vi "Send.vi"(8 "error in":errorcluster, 11 "Block Upload Initiate in":refnum<class "Block Upload Initiate Transfer.lvclass">) -> (0 "error out":errorcluster, 3 "Block Upload Initiate out":refnum<class "Block Upload Initiate Transfer.lvclass">)   [LabVIEW 2020, in "CANopen.lvlib" / "SDO Manager.lvlib" / "Block Upload Initiate Transfer.lvclass"]
doc: "SDO block upload initiate (phase I)"
uses:
  Block Upload Initiate Transfer.lvclass
  D:/git/CANopen-LabVIEW/source/SDO/SDO Manager/SDO Transfer/SDO Transfer.lvclass
  Typedefs/Function Code.ctl
  SDO Transfer/SDO Transfer.lvclass/SDO Transfer.ctl
  Block Upload Initiate Transfer.lvclass/Block Upload Initiate Transfer.ctl
  CANopen Message/CANopen Message.lvclass/CANopen Message.ctl
  SDO Transfer/Get ICommunicate.vi
  SDO Transfer/Get Node-ID.vi
  SDO Transfer/Get Multiplexer.vi
  Get Block Size.vi
  Get Protocol Switch Threshold.vi
  CANopen Message/Encode COB-ID.vi
  HAL/Source/Interfaces/ICommunicate/ICommunicate.lvclass
  CANopen Message/CANopen Message.lvclass
  CANopen.lvlib
  SDO Transfer/SDO Transfer.lvclass
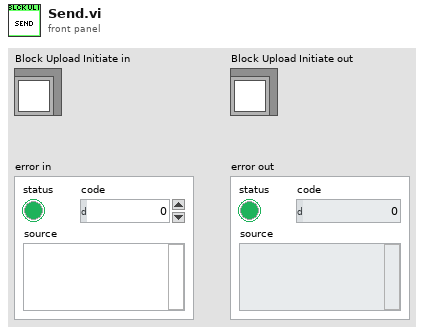
[diagram p1: front panel]
types:
  T1 = typedef "CANopen.lvlib/Function Code.ctl" = u8
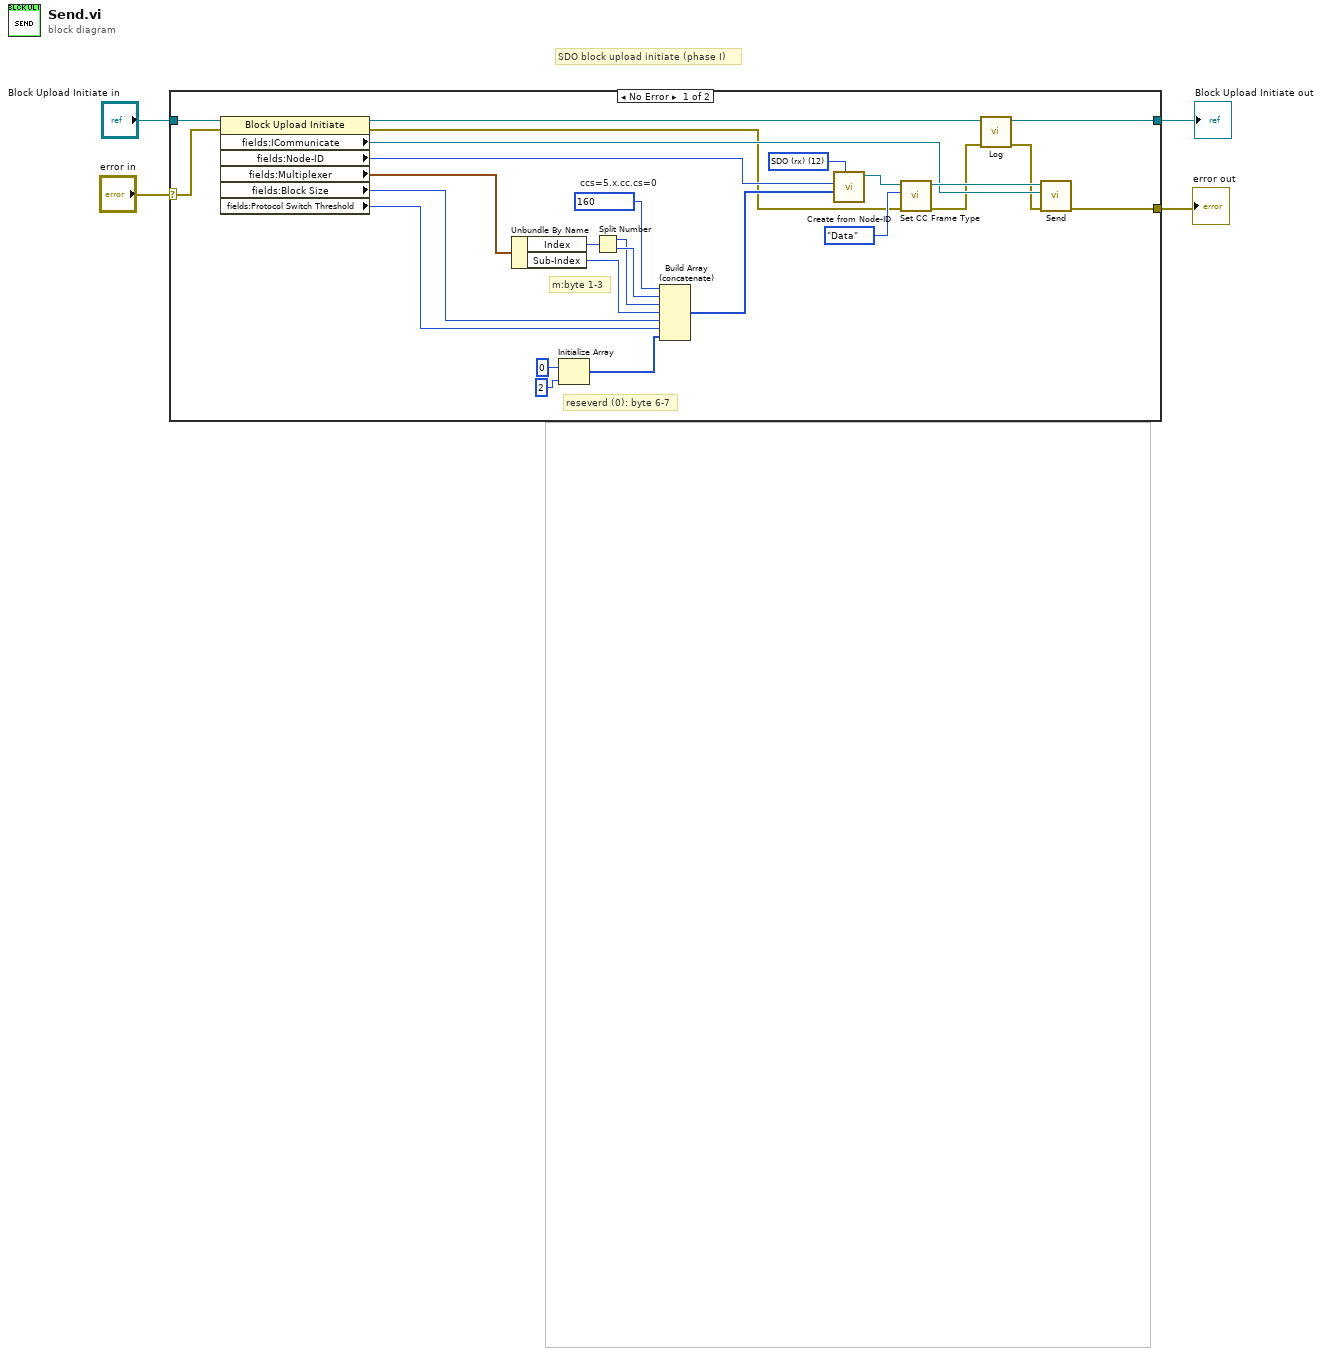
[diagram p0: block diagram]
diagram:
  # "SDO block upload initiate (phase I)"
  n1 = case shown="No Error" "error in" {
    selector: "error in" -> [w30 w31]
    tunnel: "Block Upload Initiate in" -> [w29 w32]
    tunnel: [w12 w32] -> w1
    tunnel: [w11 w31] -> w2
    frame No Error {
      w19 = T1 12 items=["NMT"=0, "EMCY/SYNC"=1, "TIME"=2, "PDO1 (tx)"=3, "PDO1 (rx)"=4, "PDO2 (tx)"=5, "PDO2 (rx)"=6, "PDO3 (tx)"=7, "PDO3 (rx)"=8, "PDO4 (tx)"=9, "PDO4 (rx)"=10, "SDO (tx)"=11, "SDO (rx)"=12, "NMT error control"=14] ("Function Code")
      w23 = u8 160  # ccs=5.x.cc.cs=0
      # "reseverd (0): byte 6-7"
      # "m:byte 1-3"
      n2 = property class="Block Upload Initiate"(reference=w29, error in=w30) -> (reference out=w13:refnum<class "Block Upload Initiate Transfer.lvclass">, error out=w10:errorcluster, "fields:ICommunicate"=w14:refnum<class "ICommunicate.lvclass">, "fields:Node-ID"=w28:u8, "fields:Multiplexer"=w21:cluster{"Index":u16, "Sub-Index":u8}, "fields:Block Size"=w6:u8, "fields:Protocol Switch Threshold"=w5:u8)
      n3 = Unbundle By Name(w21) -> ("Index"=w27:u16, "Sub-Index"=w24:u8)
      n4 = Initialize Array(u8 0, 2 ("y")) -> (w7:u8[])
      n5 = Split Number(x=w27) -> (hi(x)=w25:u8, lo(x)=w26:u8)
      n6 = Build Array (concatenate)(w23, w26, w25, w24, w6, w5, w7) -> (w20:u8[])
      n7 = call "Create from Node-ID.vi"("Function Code"=w19, "Data"=w20, "Node-ID"=w28) -> ("CANopen Message"=w18:refnum<class "CANopen Message.lvclass">)  [unwired: 8 in]
      n8 = call "Set CC Frame Type.vi"("error in"=w10, "CC Frame Type"=enum8{"Data", "Remote", "Error", "Overload"}."Data", "CANopen Message in"=w18) -> ("error out"=w9:errorcluster, "CANopen Message out"=w17:refnum<class "CANopen Message.lvclass">)  [unwired: 7 in]
      n9 = call "Log.vi"("error in"=w9, "SDO Transfer in"=w13) -> ("error out"=w8:errorcluster, "SDO Transfer out"=w12:refnum<class "Block Upload Initiate Transfer.lvclass">)  [unwired: 8 in]
      n10 = call "Send.vi"("error in"=w8, "ICommunicate"=w14, "CANopen Message in"=w17) -> ("error out"=w11:errorcluster)  [unwired: 7 in, 1 out]
    }
    frame Error {
    }
  }
  "Block Upload Initiate out" <- w1
  "error out" <- w2
